vi "Go to next Coordinate (Keith Koch's conflicted copy 2013-05-10).vi"() -> (0 "Reached/Missed":bool)   [LabVIEW 2011]
uses:
  _GlobalVariables&Libraries/ATV Program Global Variables.vi
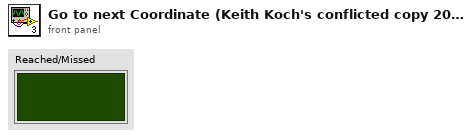
[diagram p1: front panel]
types:
  T1 = cluster{"Navigation Coordinates":cluster{"Latitude":dbl, "Longitude":dbl}[], "Coordinate Count":u32, "Drive Speed":string, "Steer Angle":dbl, "Steering":dbl, "Direction to next Coordinate":dbl, "Drive":dbl, "Navigation Path":string}
  T2 = cluster{"GPS VISA resource name":refnum<visa-resource-name>, "GPS Error":errorcluster, "Disable GPS VISA":bool, "Latitude":dbl, "Longitude":dbl, "Latitude Uncertainty":dbl, "Longitude Uncertainty":dbl, "GPS Signal":u32}
  T3 = cluster{"Obstacle Detected":bool, "Drive Speed":string, "Steer Angle":string, "Left Object":bool, "Right Object":bool, "Center Object":bool, "Rear Left":bool, "Rear Right":bool}
  T4 = cluster{"End ATV Program":bool, "E-Stop":bool, "Save Logfile":bool, "Logfile Iteration Delay (ms)":u32, "Loop iteration time (ms)":u32, "Logfile Location":path, "Default GPS Navigation Path":path, "Computer":string, "Default GPS Boundary Path":path}
  T5 = cluster{"Drive Value Output String":string, "Steer Value Output String":string, "Error Out":errorcluster, "Initial Encoder Counts":string, "Disable Galil Terminal":bool, "Command Input":string}
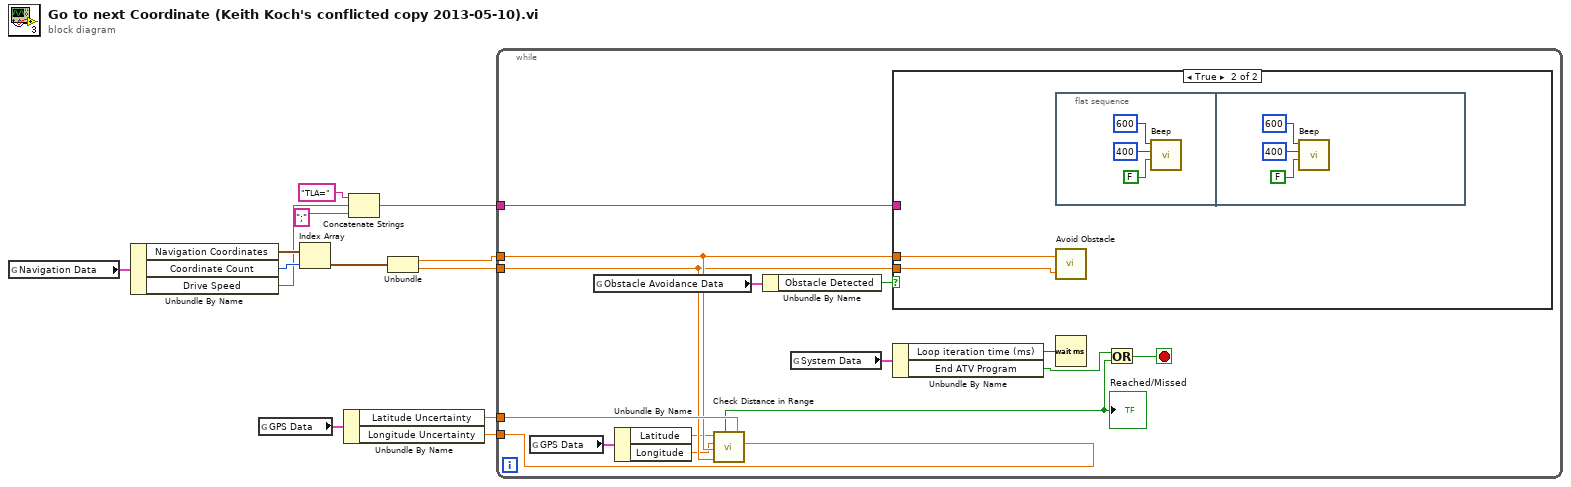
[diagram p0: block diagram]
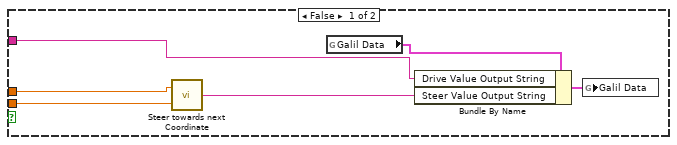
[diagram p2: hidden frame]
diagram:
  n1 = global read "ATV Program Global Variables.vi" "Navigation Data"() -> (w13:T1)
  n2 = Unbundle By Name(w13) -> ("Navigation Coordinates"=w12:cluster{"Latitude":dbl, "Longitude":dbl}[], "Coordinate Count"=w11:u32, "Drive Speed"=w2:string)
  n3 = global read "ATV Program Global Variables.vi" "GPS Data"() -> (w7:T2)
  n4 = Index Array(array=w12, index=w11) -> (element=w10:cluster{"Latitude":dbl, "Longitude":dbl})
  n5 = Unbundle By Name(w7) -> ("Latitude Uncertainty"=w5:dbl, "Longitude Uncertainty"=w6:dbl)
  n6 = Concatenate Strings("TLA=" ("string"), w2, ";" ("string")) -> (w1:string)
  n7 = Unbundle(w10) -> ("Latitude"=w9:dbl, "Longitude"=w8:dbl)
  n8 = while {
    tunnel: w9 -> [w21]
    tunnel: w8 -> [w20]
    tunnel: w6 -> [w26]
    tunnel: w1 -> [w25]
    tunnel: w5 -> [w22]
    stop <- w16 stop-if-true
    n9 = global read "ATV Program Global Variables.vi" "GPS Data"() -> (w19:T2)
    n10 = global read "ATV Program Global Variables.vi" "Obstacle Avoidance Data"() -> (w24:T3)
    n11 = Unbundle By Name(w19) -> ("Latitude"=w18:dbl, "Longitude"=w17:dbl)
    n12 = call "Check Distance in Range.vi"("Longitude Uncertainty"=w26, "Latitude Uncertainty"=w22, "Destination Longitude"=w20, "Destination Latitude"=w21, "Current Longitude"=w17, "Current Latitude"=w18) -> ("Distance in Range?"=w15:bool)  [unwired: 2 out]
    "Reached/Missed" <- w15
    n13 = Unbundle By Name(w24) -> ("Obstacle Detected"=w23:bool)
    n14 = global read "ATV Program Global Variables.vi" "System Data"() -> (w28:T4)
    n15 = case shown="True" w23 {
      tunnel: w25 -> [w29 _]
      tunnel: w21 -> [w31 w36]
      tunnel: w20 -> [w30 w35]
      frame False {
        n16 = call "Steer towards next Coordinate.vi"("Destination Longitude"=w30, "Destination Latitude"=w31) -> ("Steer Value Output String"=w32:string)
        n17 = global read "ATV Program Global Variables.vi" "Galil Data"() -> (w33:T5)
        n18 = Bundle By Name(cluster=w33, "Drive Value Output String"=w29, "Steer Value Output String"=w32) -> (w34:T5)
        n19 = global write "ATV Program Global Variables.vi" "Galil Data"(w34) -> ()
      }
      frame True {
        n20 = flat-sequence {
          frame #0 {
            n21 = call <vilib>:"Beep.vi"("use system alert? (T)"=FALSE, "duration (msec)"=u32 400, "frequency (Hz)"=u32 600) -> ()  [unwired: 9 in]
          }
          frame #1 {
            n22 = call <vilib>:"Beep.vi"("use system alert? (T)"=FALSE, "duration (msec)"=u32 400, "frequency (Hz)"=u32 600) -> ()  [unwired: 9 in]
          }
        }
        n23 = call "Avoid Obstacle.vi"("Destination Longitude"=w35, "Destination Latitude"=w36) -> ()
      }
    }
    n24 = Unbundle By Name(w28) -> ("Loop iteration time (ms)"=w27:u32, "End ATV Program"=w14:bool)
    n25 = Wait (ms)(milliseconds to wait=w27) -> ()  [unwired: 1 out]
    n26 = Or(x=w14, y=w15) -> (x .or. y?=w16:bool)
  }
